vi "SetAOs.vi"(0 "FPGA API in":refnum<class "FPGA API Mock.lvclass">, 5 "ao":dbl[](array[numeric]), 11 "error in (no error)":errorcluster) -> (4 "FPGA API out":refnum<class "FPGA API Mock.lvclass">, 15 "error out":errorcluster)   [LabVIEW 2019, in "FPGA API Mock.lvclass"]
uses:
  FPGA API Mock.lvclass
  FPGA API Mock.lvclass/FPGA API Mock.ctl
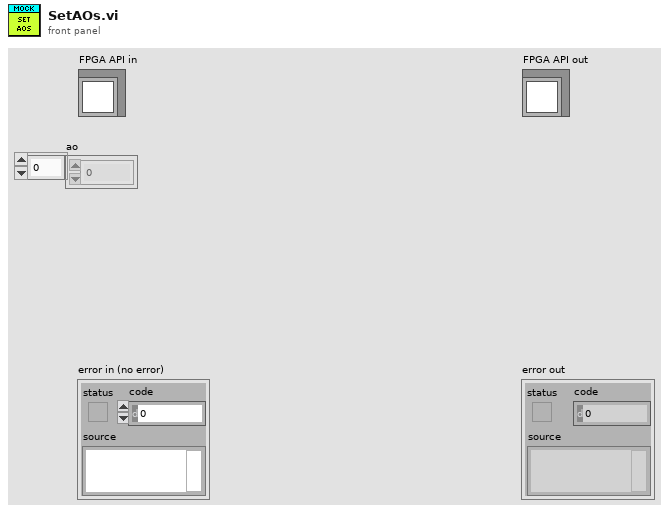
[diagram p1: front panel]
types:
  T1 = typedef "FPGA API Mock.lvclass/Data.ctl" = cluster{"DO":bool[], "DI":bool[], "AI":dbl[], "AO":dbl[]}
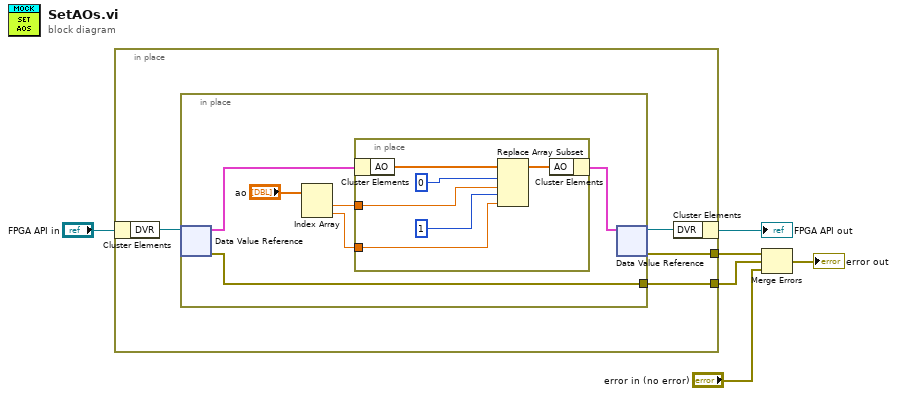
[diagram p0: block diagram]
diagram:
  n1 = in-place {
    in-place-border: [w8] -> w2
    in-place-border: [w7] -> w1
    n2 = in-place-cluster #1("FPGA API in") -> ("DVR"=w9:refnum<data-value>)
    n3 = in-place {
      in-place-border: [w11] -> w7
      n4 = in-place-dvr #2(w9) -> (w13:T1, w11:errorcluster)
      n5 = Index Array(array="ao") -> (element #1=w15:dbl, element #2=w16:dbl)  [unwired: 2 in]
      n6 = in-place {
        in-place-border: w15 -> [w20]
        in-place-border: w16 -> [w19]
        n7 = in-place-cluster #3(w13) -> ("AO"=w22:dbl[])
        n8 = Replace Array Subset(array=w22, new element #1=w20, index #1=0 ("index"), new element #2=w19, index #2=1 ("index")) -> (w21:dbl[])
        n9 = in-place-cluster #3("AO"=w21) -> (w12:T1)
      }
      n10 = in-place-dvr #2(w12) -> (w10:refnum<data-value>, w8:errorcluster)
    }
    n11 = in-place-cluster #1("DVR"=w10) -> (→"FPGA API out":refnum<class "FPGA API Mock.lvclass">)
  }
  n12 = Merge Errors(w2, w1, "error in (no error)") -> (→"error out":errorcluster)
